vi "ClearSpecificError.vi"(8 "error in":errorcluster, 11 "code":i32) -> (0 "error out":errorcluster, 2 "error cleared?":bool)   [LabVIEW 2013, in "NISE_CEF_TreeControl.lvlib"]
doc: "Clears the Error if it matches the specific code"
uses:
  NISE_CEF_TreeControl.lvlib
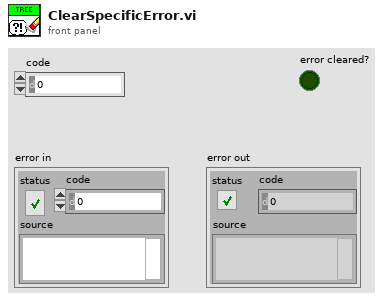
[diagram p1: front panel]
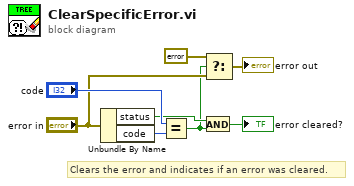
[diagram p0: block diagram]
diagram:
  # "Clears the error and indicates if an error was cleared."
  n1 = Unbundle By Name("error in") -> ("status"=w3:bool, "code"=w7:i32)
  n2 = Equal?(x="code", y=w7) -> (x = y?=w2:bool)
  n3 = And(x=w3, y=w2) -> (x .and. y?=→"error cleared?":bool)
  n4 = Select(t=errorcluster {"status"=FALSE, "code"=0, "source"=""}, s=w2, f="error in") -> (s? t:f=→"error out":errorcluster)
